vi "J-KEM_V2.vi"(10 "info in":T2) -> (0 "Temp (C)":dbl, 1 "String data out":string, 2 "info out":T1, 3 "plot data out":cluster{"Numeric Control":dbl})   [LabVIEW 2014]
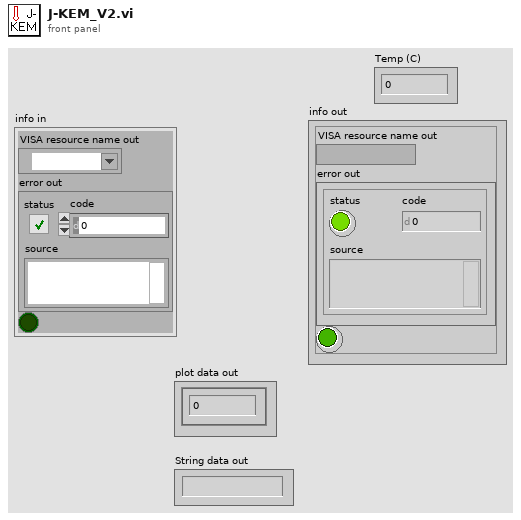
[diagram p1: front panel]
types:
  T1 = cluster{"VISA resource name out":refnum<visa-resource-name>, "error out":errorcluster, "Boolean":bool}
  T2 = cluster{"VISA resource name out":refnum<visa-resource-name>, "error out":errorcluster, bool}
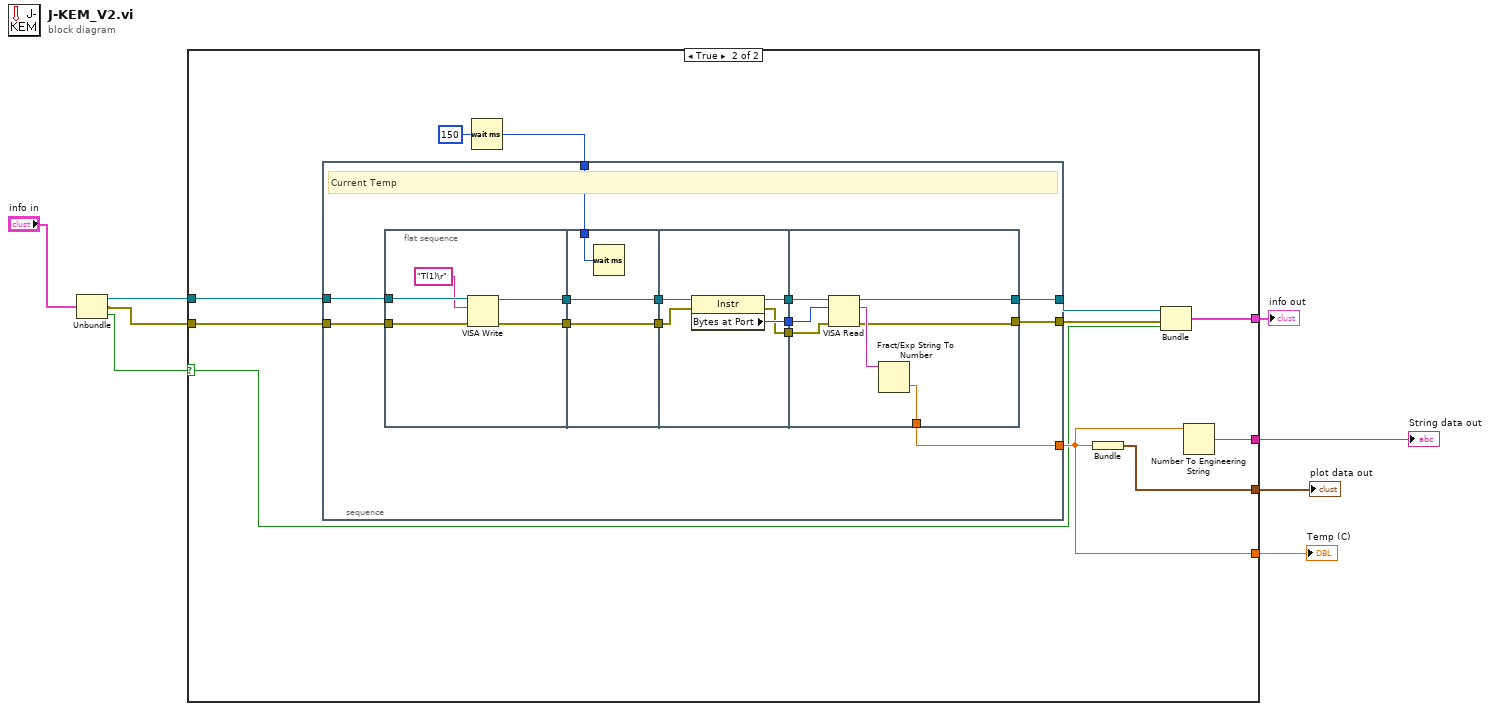
[diagram p0: block diagram]
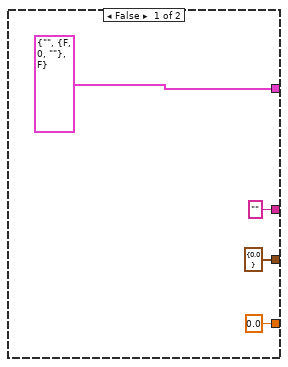
[diagram p2: hidden frame]
diagram:
  n1 = Unbundle("info in") -> ("VISA resource name out"=w4:refnum<visa-resource-name>, "error out"=w3:errorcluster, w2:bool)
  n2 = case shown="True" w2 {
    selector: w2 -> [_ w14]
    tunnel: [cluster{dbl} {0.0} w22] -> w8
    tunnel: ["" w21] -> w7
    tunnel: [0.0 w17] -> w6
    tunnel: w4 -> [_ w16]
    tunnel: w3 -> [_ w15]
    tunnel: [T2 {"VISA resource name out"="", "error out"={"status"=FALSE, "code"=0, "source"=""}, FALSE} w13] -> w1
    frame False {
    }
    frame True {
      w20 = u32 150 ("milliseconds to wait")
      n3 = stacked-sequence {
        tunnel: w16 -> [w28]
        tunnel: w15 -> [w27]
        tunnel: w20 -> [w26]
        tunnel: [w24] -> w18
        tunnel: [w23] -> w19
        tunnel: [w25] -> w17
        frame #0 {
          # "Current Temp"
          n4 = flat-sequence {
            tunnel: w28 -> [w40]
            tunnel: w27 -> [w39]
            tunnel: [w37] -> w35
            tunnel: [w36] -> w34
            tunnel: w26 -> [w43]
            tunnel: [w42] -> w33
            tunnel: w35 -> [w42]
            tunnel: w34 -> [w41]
            tunnel: [w41] -> w32
            tunnel: w33 -> [w48]
            tunnel: w32 -> [w47]
            tunnel: [w46] -> w31
            tunnel: [w45] -> w30
            tunnel: [w44] -> w29
            tunnel: w31 -> [w55]
            tunnel: w30 -> [w54]
            tunnel: w29 -> [w53]
            tunnel: [w50] -> w23
            tunnel: [w51] -> w24
            tunnel: [w49] -> w25
            frame #0 {
              n5 = VISA Write(VISA resource name=w40, write buffer="T(1)\r", error in (no error)=w39) -> (VISA resource name out=w37:refnum<visa-resource-name>, error out=w36:errorcluster)  [unwired: 1 out]
            }
            frame #1 {
              n6 = Wait (ms)(milliseconds to wait=w43) -> ()  [unwired: 1 out]
            }
            frame #2 {
              n7 = property class="Instr"(reference=w48, error in=w47) -> (reference out=w46:refnum<visa-resource-name>, error out=w44:errorcluster, "Bytes at Port"=w45:u32)
            }
            frame #3 {
              n8 = VISA Read(VISA resource name=w55, byte count=w54, error in (no error)=w53) -> (VISA resource name out=w51:refnum<visa-resource-name>, read buffer=w52:string, error out=w50:errorcluster)  [unwired: 1 out]
              n9 = Fract/Exp String To Number(string=w52) -> (number=w49:dbl)  [unwired: 3 in, 1 out]
            }
          }
        }
      }
      n10 = Wait (ms)(milliseconds to wait=w20) -> ()  [unwired: 1 out]
      n11 = Bundle(w17) -> (w22:cluster{dbl})  [unwired: 1 in]
      n12 = Bundle("VISA resource name out"=w18, "error out"=w19, w14) -> (w13:T2)  [unwired: 1 in]
      n13 = Number To Engineering String(4:w17) -> (0:w21:string)  [unwired: 3 in]
    }
  }
  "plot data out" <- w8
  "String data out" <- w7
  "Temp (C)" <- w6
  "info out" <- w1
